vi "RT_Main.vi"() -> (2 "running":bool)   [LabVIEW 2018]
uses:
  <vilib>/FPGAPlugInAG/myRIO-1900/niLvFpga_Open_myRIO-1900.vi
  <vilib>/rvi/interface/common/dynamic/niFpgaDynamicAddResources.vi
  <vilib>/Utility/error.llb/Error Cluster From Error Code.vi
  <vilib>/rvi/errors/niLvFpgaAdjustHostInterfaceError.vi
  <vilib>/rvi/interface/common/niFpgaWaitOnOcc.vi
  <vilib>/FPGAPlugInAG/Dynamic/niLvFpga_Close_Dynamic.vi
  <vilib>/rvi/interface/nirviOpenFPGA/nirviOpenFPGA.xnode
  FPGA Bitfiles/FPGAPLL_FPGATarget_FPGAMain_AD72XMDW9Sg.lvbitx
  FPGA_Main.vi
  <vilib>/rvi/interface/nirviReadWriteControl/nirviReadWriteControl.xnode
  <vilib>/rvi/interface/nirviMethod/nirviMethod.xnode
  <vilib>/rvi/interface/nirviCloseFPGA/nirviCloseFPGA.xnode
  <vilib>/rvi/errors/niLvFpgaMergeErrorWithErrorCode.vi
  <vilib>/FPGAPlugInAG/Dynamic/niLvFpga_ReadFifo_Dynamic.vi
  <vilib>/FPGAPlugInAG/Dynamic/niLvFpga_ConfigureFifo_Dynamic.vi
  <vilib>/FPGAPlugInAG/Dynamic/niLvFpga_StartFifo_Dynamic.vi
  NiFpgaLv.dll
  <vilib>/rvi/interface/Simulation/niFpgaSimulationCallBeginRW.vi
panel:
  out "size(s)":i32
  out "error fifo\nread data":errorcluster
  out "#element left":u32
  out "#elements":u32
  out "error fifo start":errorcluster
  out "error fifo \ncheck #E":errorcluster
  out "error ref":errorcluster
  out "error closing":errorcluster
  out "error fifo config":errorcluster
  out "Actual Depth":u32
  # "RT Main"
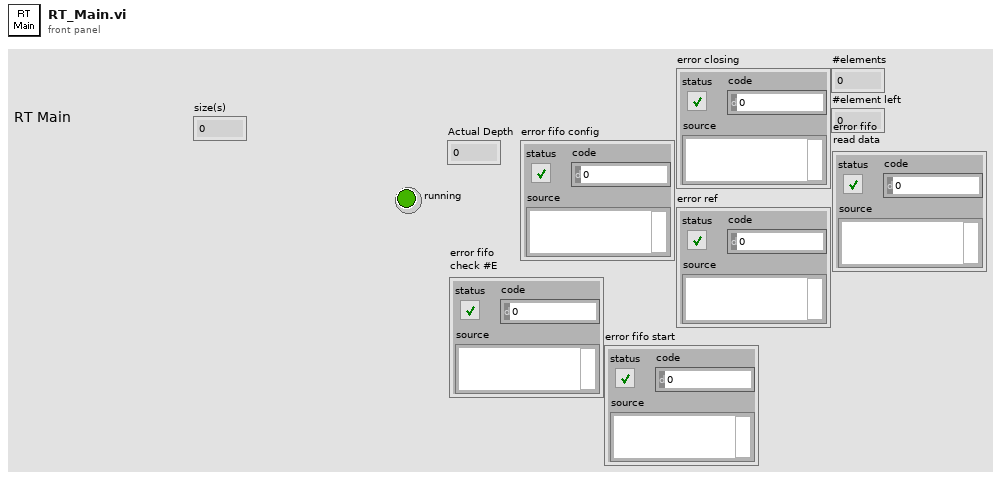
[diagram p1: front panel]
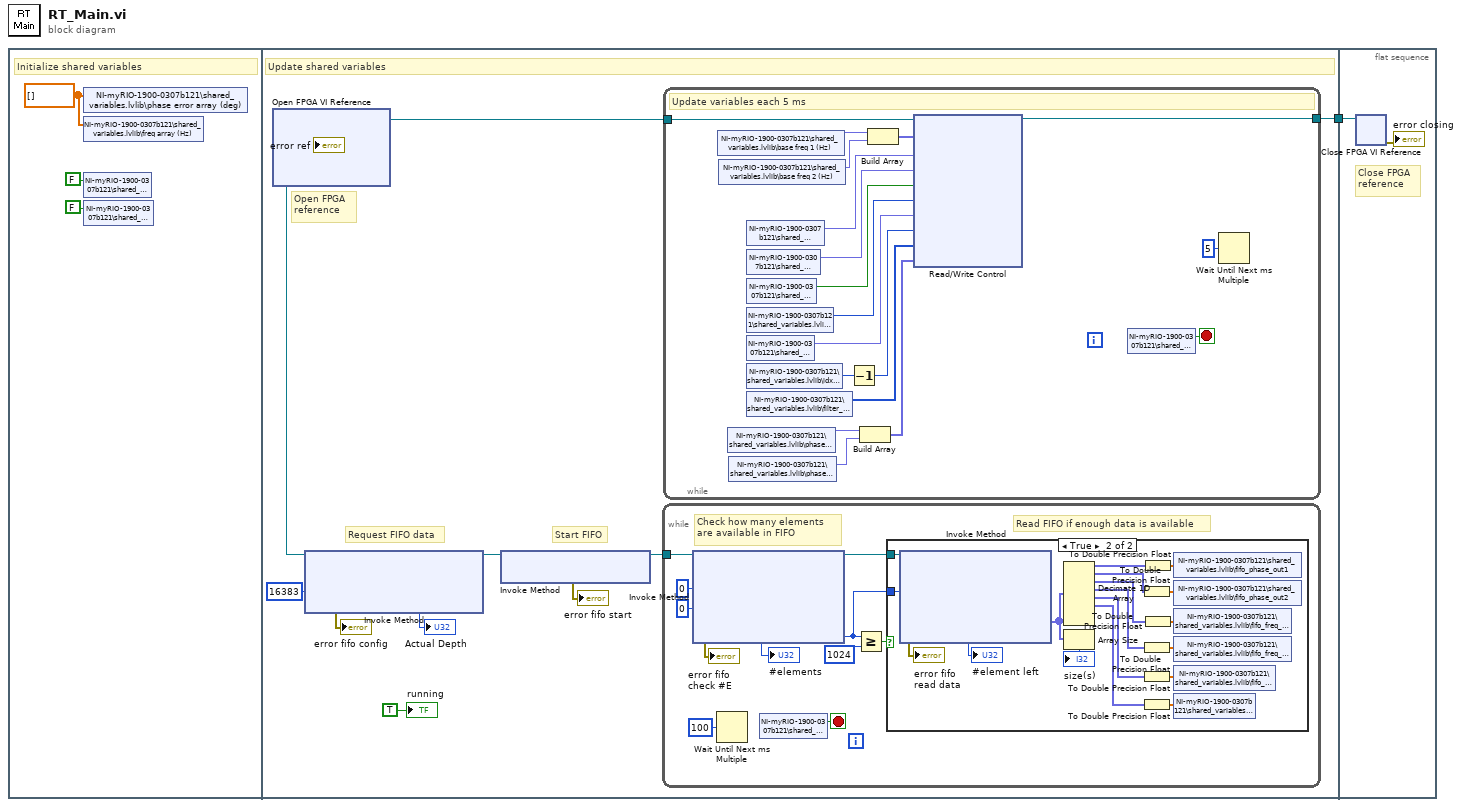
[diagram p0: block diagram]
diagram:
  n1 = flat-sequence {
    tunnel: [w13] -> w1
    tunnel: w1 -> [w62]
    frame #0 {
      w2 = dbl[] [] ("phase error array (deg)")
      # "Initialize shared variables"
      n2 = shared-variable "NI-myRIO-1900-0307b121\\shared_variables.lvlib\\phase error array (deg)"(w2) -> ()  [unwired: 1 in, 1 out]
      n3 = shared-variable "NI-myRIO-1900-0307b121\\shared_variables.lvlib\\freq array (Hz)"(w2) -> ()  [unwired: 1 in, 1 out]
      n4 = shared-variable "NI-myRIO-1900-0307b121\\shared_variables.lvlib\\stop"(FALSE ("stop")) -> ()  [unwired: 1 in, 1 out]
      n5 = shared-variable "NI-myRIO-1900-0307b121\\shared_variables.lvlib\\reset"(FALSE ("reset")) -> ()  [unwired: 1 in, 1 out]
    }
    frame #1 {
      # "Start FIFO"
      # "Request FIFO data"
      # "Open FPGA\nreference"
      # "Update shared variables"
      n6 = xnode "Open FPGA VI Reference"() -> ("FPGA VI Reference Out"=w12:refnum<k20>, "error out"=→"error ref":errorcluster)  [unwired: 2 in]
      n7 = xnode "Invoke Method"("FPGA VI Reference In"=w12, "Requested Depth"=u32 16383) -> ("FPGA VI Reference Out"=w7:refnum<k20>, "error out"=→"error fifo config":errorcluster, "Actual Depth"=→"Actual Depth":u32)  [unwired: 1 in]
      n8 = xnode "Invoke Method"("FPGA VI Reference In"=w7) -> ("FPGA VI Reference Out"=w5:refnum<k20>, "error out"=→"error fifo start":errorcluster)  [unwired: 1 in]
      n9 = while {
        tunnel: w5 -> [w23]
        stop <- w24 stop-if-true
        # "Read FIFO if enough data is available"
        # "Check how many elements\nare available in FIFO"
        n10 = xnode "Invoke Method"("FPGA VI Reference In"=w23, "Number of Elements"=u32 0, "Timeout (ms)"=0) -> ("FPGA VI Reference Out"=w18:refnum<k20>, "error out"=→"error fifo \ncheck #E":errorcluster, "Elements Remaining"=w16:u32)  [unwired: 1 in, 1 out]
        "#elements" <- w16
        n11 = Wait Until Next ms Multiple(millisecond multiple=u32 100) -> ()  [unwired: 1 out]
        n12 = shared-variable "NI-myRIO-1900-0307b121\\shared_variables.lvlib\\stop"() -> (w24:bool)  [unwired: 1 in, 1 out]
        n13 = Greater Or Equal?(x=w16, y=u32 1024) -> (x >= y?=w15:bool)
        n14 = case shown="True" w15 {
          tunnel: w18 -> [_ w42]
          tunnel: w16 -> [_ w37]
          frame False {
          }
          frame True {
            n15 = xnode "Invoke Method"("FPGA VI Reference In"=w42, "Number of Elements"=w37) -> ("error out"=→"error fifo\nread data":errorcluster, "Data"=w35:fxp<+/-,17,1>[], "Elements Remaining"=→"#element left":u32)  [unwired: 2 in, 1 out]
            n16 = Decimate 1D Array(w35) -> (w34:fxp<+/-,17,1>[], w33:fxp<+/-,17,1>[], w28:fxp<+/-,17,1>[], w27:fxp<+/-,17,1>[], w26:fxp<+/-,17,1>[], w25:fxp<+/-,17,1>[])  [unwired: 2 out]
            n17 = Array Size(array=w35) -> (size(s)=→"size(s)":i32)
            n18 = To Double Precision Float(number=w33) -> (double precision float=w36:dbl[])
            n19 = To Double Precision Float(number=w27) -> (double precision float=w32:dbl[])
            n20 = To Double Precision Float(number=w26) -> (double precision float=w30:dbl[])
            n21 = To Double Precision Float(number=w25) -> (double precision float=w29:dbl[])
            n22 = To Double Precision Float(number=w34) -> (double precision float=w39:dbl[])
            n23 = To Double Precision Float(number=w28) -> (double precision float=w31:dbl[])
            n24 = shared-variable "NI-myRIO-1900-0307b121\\shared_variables.lvlib\\fifo_phase_out1"(w39) -> ()  [unwired: 1 in, 1 out]
            n25 = shared-variable "NI-myRIO-1900-0307b121\\shared_variables.lvlib\\fifo_phase_out2"(w36) -> ()  [unwired: 1 in, 1 out]
            n26 = shared-variable "NI-myRIO-1900-0307b121\\shared_variables.lvlib\\fifo_freq_out1"(w31) -> ()  [unwired: 1 in, 1 out]
            n27 = shared-variable "NI-myRIO-1900-0307b121\\shared_variables.lvlib\\fifo_freq_out2"(w32) -> ()  [unwired: 1 in, 1 out]
            n28 = shared-variable "NI-myRIO-1900-0307b121\\shared_variables.lvlib\\fifo_adc_in"(w30) -> ()  [unwired: 1 in, 1 out]
            n29 = shared-variable "NI-myRIO-1900-0307b121\\shared_variables.lvlib\\fifo_ref"(w29) -> ()  [unwired: 1 in, 1 out]
          }
        }
      }
      n30 = while {
        tunnel: w12 -> [w60]
        tunnel: [w55] -> w13
        stop <- w54 stop-if-true
        # "Update variables each 5 ms"
        n31 = shared-variable "NI-myRIO-1900-0307b121\\shared_variables.lvlib\\base freq 1 (Hz)"() -> (w51:fxp<+/-,64,32>)  [unwired: 1 in, 1 out]
        n32 = shared-variable "NI-myRIO-1900-0307b121\\shared_variables.lvlib\\base freq 2 (Hz)"() -> (w50:fxp<+/-,64,32>)  [unwired: 1 in, 1 out]
        n33 = shared-variable "NI-myRIO-1900-0307b121\\shared_variables.lvlib\\phase_corr1"() -> (w45:fxp<+/-,64,32>)  [unwired: 1 in, 1 out]
        n34 = shared-variable "NI-myRIO-1900-0307b121\\shared_variables.lvlib\\phase_corr2"() -> (w44:fxp<+/-,64,32>)  [unwired: 1 in, 1 out]
        n35 = shared-variable "NI-myRIO-1900-0307b121\\shared_variables.lvlib\\P gain"() -> (w58:fxp<+/-,64,32>)  [unwired: 1 in, 1 out]
        n36 = shared-variable "NI-myRIO-1900-0307b121\\shared_variables.lvlib\\I gain"() -> (w57:fxp<+/-,64,32>)  [unwired: 1 in, 1 out]
        n37 = shared-variable "NI-myRIO-1900-0307b121\\shared_variables.lvlib\\reset"() -> (w56:bool)  [unwired: 1 in, 1 out]
        n38 = shared-variable "NI-myRIO-1900-0307b121\\shared_variables.lvlib\\idx_pick"() -> (w53:u8)  [unwired: 1 in, 1 out]
        n39 = shared-variable "NI-myRIO-1900-0307b121\\shared_variables.lvlib\\gain"() -> (w49:fxp<+,20,8>)  [unwired: 1 in, 1 out]
        n40 = shared-variable "NI-myRIO-1900-0307b121\\shared_variables.lvlib\\idx_scope"() -> (w48:u8)  [unwired: 1 in, 1 out]
        n41 = shared-variable "NI-myRIO-1900-0307b121\\shared_variables.lvlib\\filter_coeffs"() -> (w46:i32[])  [unwired: 1 in, 1 out]
        n42 = Decrement(x=w48) -> (x-1=w47:u8)
        n43 = Build Array(w45, w44) -> (w43:fxp<+/-,64,32>[])
        n44 = Build Array(w51, w50) -> (w52:fxp<+/-,64,32>[])
        n45 = xnode "Read/Write Control"("FPGA VI Reference In"=w60, "base freqs"=w52, "P gain"=w58, "I gain"=w57, "reset"=w56, "idx pick"=w53, "gain"=w49, "idx scope"=w47, "Filter coeffs"=w46, "phase_correction"=w43) -> ("FPGA VI Reference Out"=w55:refnum<k20>)  [unwired: 1 in, 1 out]
        n46 = shared-variable "NI-myRIO-1900-0307b121\\shared_variables.lvlib\\stop"() -> (w54:bool)  [unwired: 1 in, 1 out]
        n47 = Wait Until Next ms Multiple(millisecond multiple=u32 5) -> ()  [unwired: 1 out]
      }
      "running" <- TRUE ("running")
    }
    frame #2 {
      # "Close FPGA\nreference"
      n48 = xnode "Close FPGA VI Reference"("FPGA VI Reference In"=w62) -> ("error out"=→"error closing":errorcluster)  [unwired: 1 in]
    }
  }
